vi "Edit Status Indicator.vi"(8 "error in (no error)":errorcluster, 9 "State":T2, 11 "Instrument Status Refnum":refnum<vi>[](array[refnum])) -> (0 "error out":errorcluster)   [LabVIEW 2014]
uses:
  Instrument Status State.ctl
  Instrument Status.ctl
panel:
  out "Instrument Status":T1
  # "LICENSED MATERIALS – PROPERTY OF IBM\nCopyright IBM Corp. 2016,\nALL RIGHTS RESERVED"
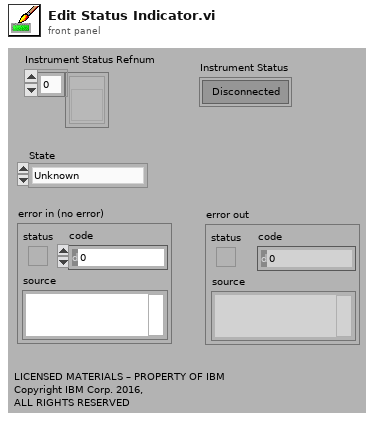
[diagram p1: front panel]
types:
  T1 = typedef "Instrument Status.ctl" = bool
  T2 = typedef "Instrument Status State.ctl" = enum16{"Unknown", "Idle", "Standby", "Configuring", "Measuring", "Moving", "Disconnected"}
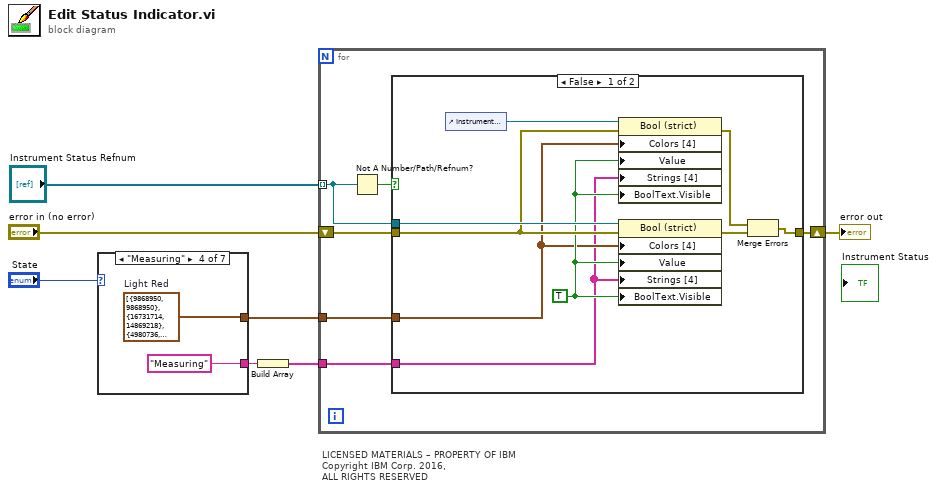
[diagram p0: block diagram]
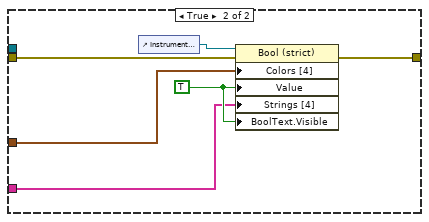
[diagram p2: hidden frame]
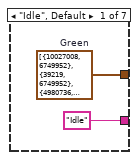
[diagram p3: hidden frame]
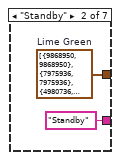
[diagram p4: hidden frame]
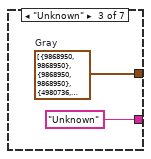
[diagram p5: hidden frame]
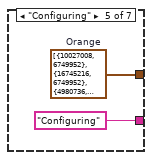
[diagram p6: hidden frame]
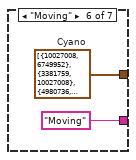
[diagram p7: hidden frame]
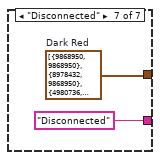
[diagram p8: hidden frame]
diagram:
  # "LICENSED MATERIALS – PROPERTY OF IBM\nCopyright IBM Corp. 2016,\nALL RIGHTS RESERVED"
  n1 = case shown="\"Measuring\"" "State" {
    tunnel: [w8 w10 w12 w14 w17 w19 w20] -> w4
    tunnel: ["Idle" "Standby" "Unknown" "Measuring" "Configuring" "Moving" "Disconnected"] -> w3
    frame "Idle", Default {
      w8 = cluster{u32, u32}[] [{10027008, 6749952}, {39219, 6749952}, {4980736, 3374848}, {19481, 3374848}]  # Green
    }
    frame "Standby" {
      w10 = cluster{u32, u32}[] [{9868950, 9868950}, {7975936, 7975936}, {4980736, 3374848}, {3955200, 3955200}]  # Lime Green
    }
    frame "Unknown" {
      w12 = cluster{u32, u32}[] [{9868950, 9868950}, {9868950, 9868950}, {4980736, 3374848}, {4934475, 5855577}]  # Gray
    }
    frame "Measuring" {
      w14 = cluster{u32, u32}[] [{9868950, 9868950}, {16731714, 14869218}, {4980736, 3374848}, {8333089, 7434609}]  # Light Red
    }
    frame "Configuring" {
      w17 = cluster{u32, u32}[] [{10027008, 6749952}, {16745216, 6749952}, {4980736, 3374848}, {8339712, 3374848}]  # Orange
    }
    frame "Moving" {
      w19 = cluster{u32, u32}[] [{10027008, 6749952}, {3381759, 10027008}, {4980736, 3374848}, {1657983, 4980736}]  # Cyano
    }
    frame "Disconnected" {
      w20 = cluster{u32, u32}[] [{9868950, 9868950}, {8978432, 9868950}, {4980736, 3374848}, {4456448, 4934475}]  # Dark Red
    }
  }
  n2 = Build Array(w3) -> (w2:string[])
  n3 = for {
    tunnel: w4 -> [w24]
    tunnel: w2 -> [w23]
    tunnel: "Instrument Status Refnum" -> [w22] mode=indexing
    shift-right: [w26] -> w6
    shift-left: "error in (no error)" -> [w27]
    n4 = Not A Number/Path/Refnum?(number/path/refnum=w22) -> (NaN/Path/Refnum?=w25:bool)
    n5 = case shown="False" w25 {
      tunnel: w22 -> [w35 _]
      tunnel: w27 -> [w33 w41]
      tunnel: [w31 w39] -> w26
      tunnel: w24 -> [w29 w38]
      tunnel: w23 -> [w28 w37]
      frame False {
        w32 = TRUE ("Value")
        n6 = control-ref of="Instrument Status"() -> (w34:refnum<vi>)
        n7 = property class="Bool (strict)"(reference=w34, error in=w33, "Colors [4]"=w29, "Value"=w32, "Strings [4]"=w28, "BoolText.Visible"=w32) -> (error out=w30:errorcluster)  [unwired: 1 out]
        n8 = property class="Bool (strict)"(reference=w35, error in=w33, "Colors [4]"=w29, "Value"=w32, "Strings [4]"=w28, "BoolText.Visible"=w32) -> (error out=w36:errorcluster)  [unwired: 1 out]
        n9 = Merge Errors(w30, w36) -> (w31:errorcluster)
      }
      frame True {
        w40 = TRUE ("Value")
        n10 = control-ref of="Instrument Status"() -> (w42:refnum<vi>)
        n11 = property class="Bool (strict)"(reference=w42, error in=w41, "Colors [4]"=w38, "Value"=w40, "Strings [4]"=w37, "BoolText.Visible"=w40) -> (error out=w39:errorcluster)  [unwired: 1 out]
      }
    }
  }
  "error out" <- w6
